vi "NonBoolesch Values Reset.vi"(10 "Value aus Projekt":string, 11 "Key aus Projekt":string) -> (2 "Value aus Projekt out":string, 3 "Default Value":string)   [LabVIEW 2020, in "ConditionalDeactivation.lvlib"]
uses:
  ConditionalDeactivation.lvlib
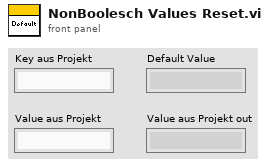
[diagram p1: front panel]
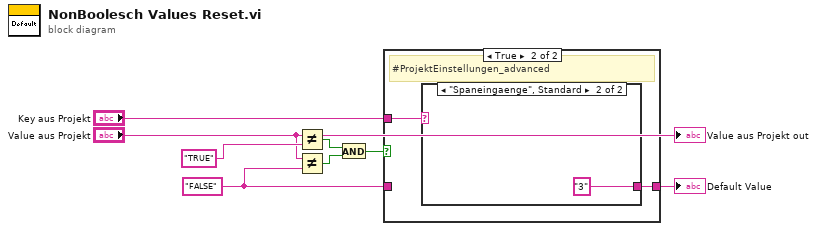
[diagram p0: block diagram]
diagram:
  w2 = "FALSE"
  n1 = Not Equal?(x="Value aus Projekt", y="TRUE") -> (x != y?=w5:bool)
  n2 = Not Equal?(x="Value aus Projekt", y=w2) -> (x != y?=w6:bool)
  n3 = And(x=w5, y=w6) -> (x .and. y?=w4:bool)
  n4 = case shown="True" w4 {
    tunnel: [w9 w10] -> w3
    tunnel: w2 -> [w9 _]
    tunnel: "Key aus Projekt" -> [_ w11]
    frame False {
    }
    frame True {
      # "#ProjektEinstellungen_advanced"
      n5 = case shown="\"Spaneingaenge\", Standard" w11 {
        tunnel: [_ "3"] -> w10
        frame "False" {
        }
        frame "Spaneingaenge", Default {
        }
      }
    }
  }
  "Default Value" <- w3
  "Value aus Projekt out" <- "Value aus Projekt"
